vi "Get Cluster SubCtl Name.vi"(8 "error in (no error)":errorcluster, 11 "Clust Ref":refnum<vi>) -> (0 "error out":errorcluster, 2 "CtlName":string[](array[string]), 3 "reference out":refnum<vi>)   [LabVIEW 2015]
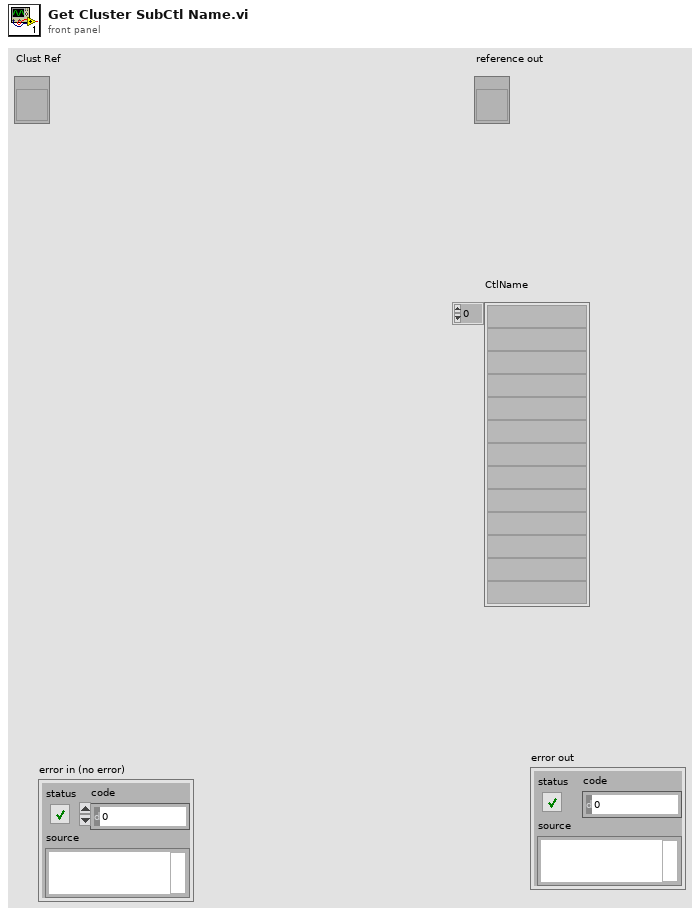
[diagram p1: front panel]
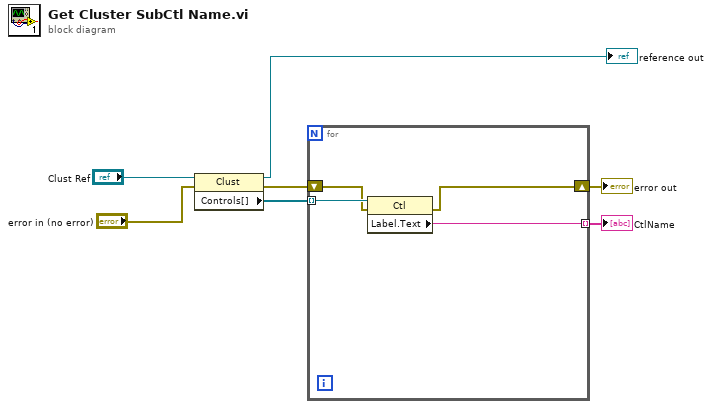
[diagram p0: block diagram]
diagram:
  n1 = property class="Clust"(reference="Clust Ref", error in="error in (no error)") -> (reference out=→"reference out":refnum<vi>, error out=w6:errorcluster, "Controls[]"=w7:refnum<vi>[])
  n2 = for {
    tunnel: w7 -> [w11] mode=indexing
    shift-right: [w9] -> w1
    shift-left: w6 -> [w10]
    tunnel: [w8] -> w5 mode=indexing
    n3 = property class="Ctl"(reference=w11, error in=w10) -> (error out=w9:errorcluster, "Label.Text"=w8:string)  [unwired: 1 out]
  }
  "CtlName" <- w5
  "error out" <- w1
